vi "Shutdown.vi"(0 "Limits File":path, 5 "Results File":path, 11 "error in":errorcluster) -> (15 "error out":errorcluster)   [LabVIEW 2024]
doc: "Fake shutdown test"
uses:
  <userlib>/_OpenG.lib/time/time.llb/openg_time.lvlib
  <userlib>/_OpenG.lib/appcontrol/appcontrol.llb/openg_application_control.lvlib
panel:
  # "Shutdown Test VI"
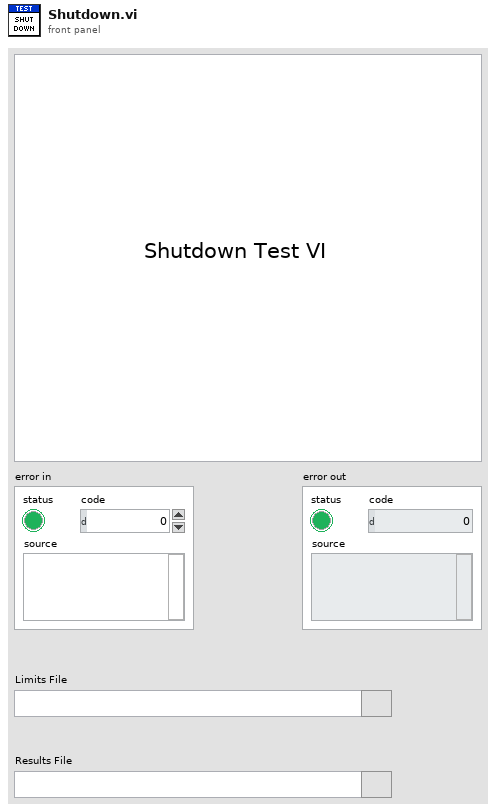
[diagram p1: front panel]
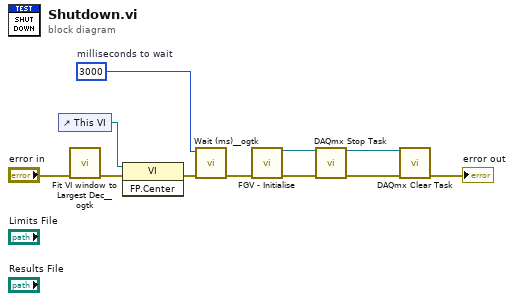
[diagram p0: block diagram]
diagram:
  w10 = u32 3000  # milliseconds to wait
  n1 = control-ref of="This VI"() -> (w7:refnum<vi>)
  n2 = call <userlib>:"Fit VI window to Largest Dec__ogtk.vi"("error in (no error)"="error in") -> ("error out"=w9:errorcluster)  [unwired: 5 in, 1 out]
  n3 = invoke class="VI" method="FP.Center"(reference=w7, error in=w9) -> (error out=w8:errorcluster)  [unwired: 1 in, 2 out]
  n4 = call <userlib>:"Wait (ms)__ogtk.vi"("error in (no error)"=w8, "milliseconds to wait"=w10) -> ("error out"=w1:errorcluster)  [unwired: 8 in, 1 out]
  n5 = call "FGV - Initialise.vi"("Error In"=w1) -> ("task out"=w3:refnum<k21>, "Error Out"=w2:errorcluster)  [unwired: 7 in, 1 out]
  n6 = call <vilib>:"DAQmx Stop Task.vi"("task/channels in"=w3, "error in"=w2) -> ("task out"=w5:refnum<k21>, "error out"=w6:errorcluster)  [unwired: 12 in]
  n7 = call <vilib>:"DAQmx Clear Task.vi"("task in"=w5, "error in"=w6) -> ("error out"=→"error out":errorcluster)  [unwired: 13 in]
